vi "Set_Bandwidth_DLPVA-Series.vi"(3 "error in":errorcluster, 4 "Status":i32, 5 "Bandwidth":enum16{"1 kHz", "100 kHz"}(ring), 6 "index":i32) -> (0 "error out":errorcluster, 1 "Status_out":i32, 2 "index_out":i32)   [LabVIEW 2013, in "FEMTO_LUCI-10.lvlib"]
doc: "This function sets the bandwidth for the selected device."
uses:
  FEMTO_LUCI-10.lvlib
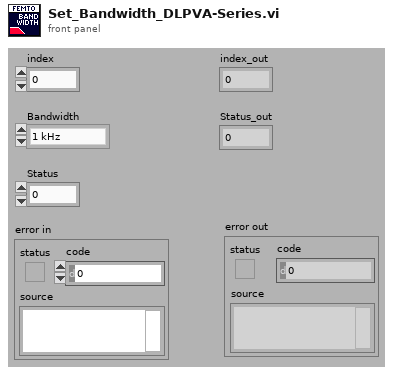
[diagram p1: front panel]
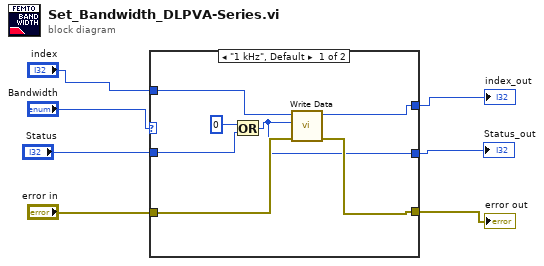
[diagram p0: block diagram]
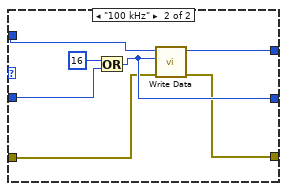
[diagram p2: hidden frame]
diagram:
  n1 = case shown="\"1 kHz\", Default" "Bandwidth" {
    tunnel: [w8 w21] -> w7
    tunnel: "Status" -> [w11 w20]
    tunnel: [w9 w19] -> w5
    tunnel: "error in" -> [w10 w18]
    tunnel: [w12 w17] -> w3
    tunnel: "index" -> [w13 w16]
    frame "1 kHz", Default {
      n2 = Or(x=0 ("data_low"), y=w11) -> (x .or. y?=w8:i32)
      n3 = call "Write Data.vi"("error in (no error)"=w10, "data_low"=w8, "index"=w13) -> ("error out"=w9:errorcluster, "index_out"=w12:i32)  [unwired: 1 in, 6 out]
    }
    frame "100 kHz" {
      n4 = Or(x=16 ("data_low"), y=w20) -> (x .or. y?=w21:i32)
      n5 = call "Write Data.vi"("error in (no error)"=w18, "data_low"=w21, "index"=w16) -> ("error out"=w19:errorcluster, "index_out"=w17:i32)  [unwired: 1 in, 6 out]
    }
  }
  "index_out" <- w3
  "error out" <- w5
  "Status_out" <- w7
